vi "XY Graph Set Plot TipStrip.vi"(4 "Top/Bottom(F)":bool, 5 "Offset (10)":i32=10, 6 "Left/Right(F)":bool, 7 "TipStrip Refnum":refnum<vi>, 8 "Error In":errorcluster, 9 "Max Length (200)":i32=200, 10 "Coords":T1, 11 "XY Graph Refnum":refnum<vi>) -> (0 "Error Out":errorcluster, 1 "Plot Name":string, 2 "Plot at Coordinates":i32)   [LabVIEW 2021, in "XY Graph Add-Ons.lvlib"]
doc: "Shows a tipstrip indicating the name of the plot in the graph legend over which the mouse is located.\n\nThe maximal length (<b>Max Length</b>)of the tipstrip is optional (default: 200 pixels).\nThe relative location of the tipstrip (with respect to the mouse) can be specified with two flags (<b>Top/Bottom</b> and <b>Left/Right</b>) and an <b>Offset</b> value.\nThe default is bottom right, with an offset of 10 pixels in both directions.\n\nIf the mouse is over a plot legend, its index and legend are returned. Otherwise -1 and an empty string are returned."
uses:
  XY Graph/XY Graph Add-Ons.lvlib
  <vilib>/Utility/miscctls.llb/LVPoint32TypeDef.ctl
  <vilib>/Utility/miscctls.llb/LVPositionTypeDef.ctl
  Get Plot at Mouse Click (XY Graph)/Get Plot at Mouse Click [AAC].vi
  Graphs.lvlib
  GUI/GUI.lvlib
  Error/Error.lvlib
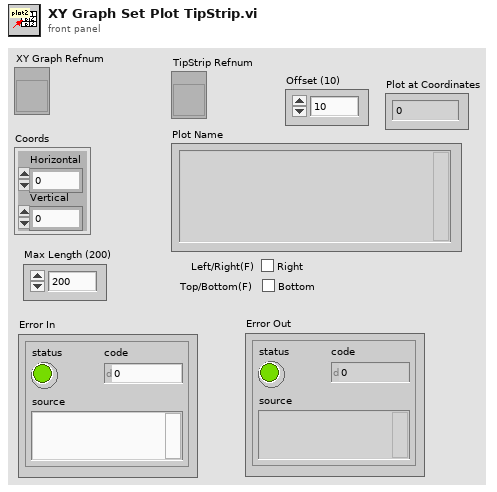
[diagram p1: front panel]
types:
  T1 = typedef "LVPoint32TypeDef.ctl" = cluster{"Horizontal":i32, "Vertical":i32}
  T2 = typedef "XY Graph Add-Ons.lvlib/XY Graph Refnum.ctl" = refnum<vi>
  T3 = typedef "LVPositionTypeDef.ctl" = cluster{"Left":i32, "Top":i32}
  T4 = typedef "LVBoundsTypeDef.ctl" = cluster{"Width":u32, "Height":u32}
  T5 = typedef "LVPointTypeDef.ctl" = cluster{"Horizontal":i16, "Vertical":i16}
  T6 = cluster{"left":i16, "top":i16, "right":i16, "bottom":i16}
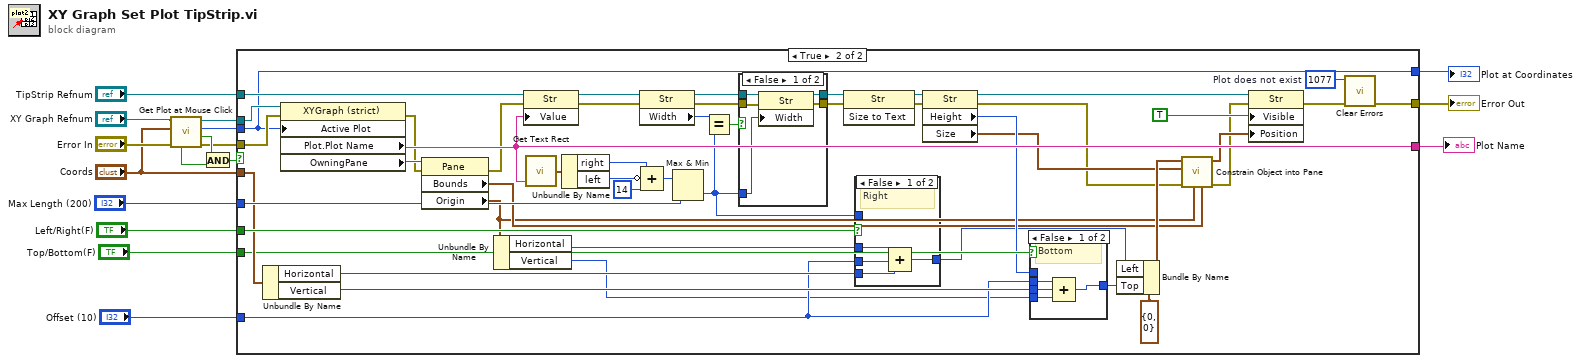
[diagram p0: block diagram]
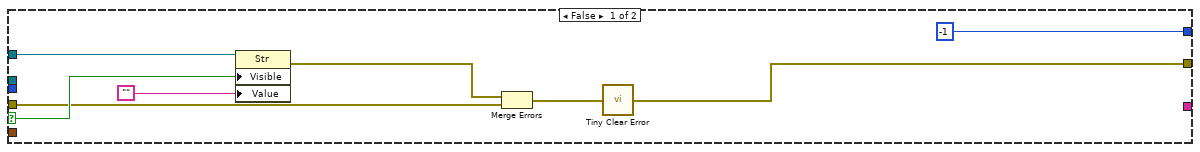
[diagram p2: hidden frame]
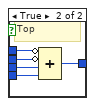
[diagram p3: hidden frame]
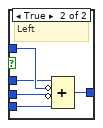
[diagram p4: hidden frame]
diagram:
  n1 = call-poly "Get Plot at Mouse Click.vi"("error in (no error)"="Error In", "Mouse Click Coordinates"="Coords", "XYGraph Ref"="XY Graph Refnum") -> ("error out"=w11:errorcluster, "Click is in Legend?"=w15:bool, "Plot at Coordinates"=w13:i32, "XYGraph Ref"=w14:T2, "Found?"=w1:bool)  [unwired: 2 in, 2 out]
  n2 = And(x=w15, y=w1) -> (x .and. y?=w2:bool)
  n3 = case shown="True" w2 {
    selector: w2 -> [w24 _]
    tunnel: w14 -> [_ w74]
    tunnel: w13 -> [_ w40]
    tunnel: "TipStrip Refnum" -> [w25 w72]
    tunnel: w11 -> [w22 w73]
    tunnel: [w18 w27] -> w10
    tunnel: "Coords" -> [_ w53]
    tunnel: [_ w67] -> w8
    tunnel: "Max Length (200)" -> [_ w55]
    tunnel: "Left/Right(F)" -> [_ w54]
    tunnel: "Top/Bottom(F)" -> [_ w52]
    tunnel: "Offset (10)" -> [_ w42]
    tunnel: [-1 ("Plot at Coordinates") w40] -> w3
    frame False {
      n4 = property class="Str"(reference=w25, "Visible"=w24, "Value"="") -> (error out=w19:errorcluster)  [unwired: 1 in, 1 out]
      n5 = Merge Errors(w19, w22) -> (w20:errorcluster)
      n6 = call "Tiny Clear Error.vi"("Error In"=w20) -> ("no Error Out"=w18:errorcluster)  [unwired: 8 in]
    }
    frame True {
      w26 = 1077  # Plot does not exist
      n7 = Unbundle By Name(w53) -> ("Horizontal"=w46:i32, "Vertical"=w51:i32)
      n8 = property class="XYGraph (strict)"(reference=w74, error in=w73, "Active Plot"=w40) -> (error out=w38:errorcluster, "Plot.Plot Name"=w67:string, "OwningPane"=w39:refnum<vi>)  [unwired: 1 out]
      n9 = property class="Pane"(reference=w39, error in=w38) -> (error out=w37:errorcluster, "Bounds"=w33:T4, "Origin"=w32:T5)  [unwired: 1 out]
      n10 = Unbundle By Name(w32) -> ("Horizontal"=w31:i16, "Vertical"=w30:i16)
      n11 = property class="Str"(reference=w72, error in=w37, "Value"=w67) -> (reference out=w69:refnum<vi>, error out=w68:errorcluster)
      n12 = call <vilib>:"Get Text Rect.vi"("text"=w67) -> ("rect"=w66:T6)  [unwired: 8 in]
      n13 = Unbundle By Name(w66) -> ("right"=w65:i16, "left"=w64:i16)
      n14 = property class="Str"(reference=w69, error in=w68) -> (reference out=w59:refnum<vi>, error out=w58:errorcluster, "Width"=w61:u32)
      n15 = Compound Arithmetic op=ADD(w65, invert w64, i16 14 ("value")) -> (w62:i16)
      n16 = Max & Min(x=w62, y=w55) -> (min(x,y)=w47:i32)  [unwired: 1 out]
      n17 = Equal?(x=w61, y=w47) -> (x = y?=w60:bool)
      n18 = case shown="False" w60 {
        tunnel: w59 -> [w97 w99]
        tunnel: w58 -> [w96 w98]
        tunnel: [w95 w99] -> w57
        tunnel: [w94 w98] -> w56
        tunnel: w47 -> [w93 _]
        frame False {
          n19 = property class="Str"(reference=w97, error in=w96, "Width"=w93) -> (reference out=w95:refnum<vi>, error out=w94:errorcluster)
        }
        frame True {
        }
      }
      n20 = invoke class="Str" method="Size to Text"(reference=w57, error in=w56) -> (reference out=w50:refnum<vi>, error out=w49:errorcluster)  [unwired: 1 in, 1 out]
      n21 = case shown="False" w54 {
        tunnel: w47 -> [_ w90]
        tunnel: w46 -> [w87 w92]
        tunnel: w42 -> [w86 w91]
        tunnel: [w85 w89] -> w41
        tunnel: w31 -> [w84 w88]
        frame False {
          # "Right"
          n22 = Compound Arithmetic op=ADD(w84, w86, w87) -> (w85:i32)
        }
        frame True {
          # "Left"
          n23 = Compound Arithmetic op=ADD(w88, invert w90, invert w91, w92) -> (w89:i32)
        }
      }
      n24 = property class="Str"(reference=w50, error in=w49) -> (reference out=w48:refnum<vi>, error out=w29:errorcluster, "Height"=w43:u32, "Size"=w34:T4)
      n25 = case shown="False" w52 {
        tunnel: w51 -> [w78 w83]
        tunnel: w42 -> [w77 w82]
        tunnel: [w76 w81] -> w44
        tunnel: w43 -> [_ w80]
        tunnel: w30 -> [w75 w79]
        frame False {
          # "Bottom"
          n26 = Compound Arithmetic op=ADD(w77, w78, w75) -> (w76:i32)
        }
        frame True {
          # "Top"
          n27 = Compound Arithmetic op=ADD(invert w80, invert w82, w83, w79) -> (w81:u32)
        }
      }
      n28 = Bundle By Name(cluster=T3 {"Left"=0, "Top"=0} ("Position"), "Left"=w41, "Top"=w44) -> (w35:T3)
      n29 = call "Constrain Object into Pane.vi"("Pane Bounds"=w33, "Panel Origin"=w32, "Error In"=w29, "Object Size"=w34, "Object Position in"=w35) -> ("Error Out"=w28:errorcluster, "Object Position out"=w36:T3)  [unwired: 5 in]
      n30 = property class="Str"(reference=w48, error in=w28, "Visible"=TRUE, "Position"=w36) -> (error out=w71:errorcluster)  [unwired: 1 out]
      n31 = call <vilib>:"Clear Errors.vi"("error in (no error)"=w71, "specific error code to clear (0: all)"=w26) -> ("error out"=w27:errorcluster)  [unwired: 4 in, 1 out]
    }
  }
  "Error Out" <- w10
  "Plot Name" <- w8
  "Plot at Coordinates" <- w3
